vi "MultiChannelfFeedbackCooling (FPGA).vi"() -> ()   [LabVIEW 2016]
doc: "This VI will read single point values from 4 channels of a R Series board at a specified rate."
uses:
  <vilib>/rvi/Emulation/niFpgaGetClockAttributes.vi
  <vilib>/rvi/Emulation/niFpgaSctlEmulationGetInTimedLoop.vi
  <vilib>/rvi/Emulation/niFpgaEmulationReportErrorSimple.vi
  <vilib>/rvi/eio/common/nirviEmuTemplateMethod_errors.vi
  <vilib>/rvi/Memory/Memory_Emulation/nirvimemoryFastEmulation.vi
  <vilib>/rvi/Memory/Memory_Emulation/nirvimemoryEmulation.vi
  <vilib>/rvi/Emulation/niFpgaEmulationIsFPGAContextNoSignature.vi
  <vilib>/rvi/DataTransferAndStorage/Container/Common/niFpgaContainerGetUniqueNameForEmu.vi
  <vilib>/rvi/Emulation/niFpgaProcessEmulError.vi
  <vilib>/rvi/errors/nirviReportUnexpectedCaseInternalError (U32).vi
  <vilib>/rvi/Memory/Memory_Emulation/niFpgaMemoryEmulationCacheClearOnFirstRun.vi
  <vilib>/rvi/Memory/Memory_Emulation/nirvimemoryEmulationManagerCache_MakeExclusive.vi
  <vilib>/rvi/Memory/Memory_Emulation/niFpgaMemoryEmulationValidateCache.vi
  <vilib>/rvi/Memory/Memory_Emulation/nirvimemoryEmulationManagerCache_InsertValue.vi
  <vilib>/Utility/error.llb/Clear Errors.vi
  <vilib>/rvi/Memory/Memory_Emulation/nirvimemoryEmulationManagerCache_ReleaseExclusive.vi
  <vilib>/rvi/Memory/Memory_Emulation/nirvimemoryEmulationManagerCache_GetValue.vi
  <vilib>/rvi/Memory/Memory_Emulation/nirvimemoryEmulationManagerCache_SetValue.vi
  <vilib>/rvi/Emulation/niFpgaSctlEmulationResourceMgr.vi
  <vilib>/rvi/Emulation/niFpgaCriticalErrorInLSC.vi
  <vilib>/eio/EIONode/EIONode.xnode
  <vilib>/rvi/DataTransferAndStorage/Container/XNode/niFpgaContainer.xnode
  <vilib>/rvi/FXPMathLib/FxpInterpret/XNode/nifxpmath_Interpret.xnode
panel:
  in  "pg_img":fxp<+/-,24,12>
  in  "dg_img":fxp<+/-,24,12>
  in  "ig_img":fxp<+/-,24,6>
  in  "setpt_img":i16
  out "AI_img":i16
  in  "lp coeff_img":i32[](array[numeric])=[1008310688, 32715568]
  in  "Upper lim_img":fxp<+/-,16,16>
  in  "Lower lim_img":fxp<+/-,16,16>
  in  "lp coeff d2":i32[](array[numeric])=[1008310688, 32715568]
  in  "hp coeff_img":i32[](array[numeric])=[946630756, 1010186290]
  out "tot_fb_img":i16
  out "fb_img":i16
  in  "output offset_img":i16
  in  "lp coeff 2":i32[](array[numeric])=[1008310688, 32715568]
  in  "data_buffer3":i16
  in  "Arb gain (ch2)":fxp<+/-,24,12>=0.5 caption="RMS"
  in  "lp coeff 0":i32[](array[numeric])=[1008310688, 32715568]
  in  "lp coeff 1":i32[](array[numeric])=[1008310688, 32715568]
  in  "hp coeff d2":i32[](array[numeric])=[946630756, 1010186290]
  in  "hp coeff 2":i32[](array[numeric])=[946630756, 1010186290]
  in  "hp coeff 1":i32[](array[numeric])=[946630756, 1010186290]
  in  "hp coeff 0":i32[](array[numeric])=[946630756, 1010186290]
  in  "Use_PID2_X 2":bool
  out "AI5":i16
  in  "Dc Pos d2":i16
  out "tot_fb_2":i16
  out "tot_fb_1":i16
  out "tot_fb_0":i16
  out "fb_d2":i16
  in  "output offset 2":i16
  in  "output offset 1":i16
  in  "output offset 0":i16
  in  "Lower lim 4":fxp<+/-,16,16>
  in  "Upper lim d0 3":fxp<+/-,16,16>
  in  "pg d0 3":fxp<+/-,24,12>
  in  "ig d03":fxp<+/-,24,6>
  in  "dg d0 3":fxp<+/-,24,12>
  out "fb_2":i16
  in  "ig 3":fxp<+/-,24,6>
  out "written_address":u32
  in  "ready_to_write":bool
  in  "Arb steps per cycle":u16
  in  "data_buffer2":i16
  in  "data_buffer_1":i16
  in  "write_address":u16
  in  "Arb gain (ch1)":fxp<+/-,24,12>=0.5 caption="RMS"
  in  "Arb gain (ch0)":fxp<+/-,24,12>=0.5 caption="RMS"
  out "fb_1":i16
  out "fb_0":i16
  in  "Dc Pos 1":i16
  in  "Dc Pos 0":i16
  in  "Lower lim 2":fxp<+/-,16,16>
  in  "Upper lim 2":fxp<+/-,16,16>
  in  "dg 2":fxp<+/-,24,12>
  in  "pg 2":fxp<+/-,24,12>
  out "AI2":i16
  in  "Dc Pos 2":i16
  out "AI1":i16
  in  "dg 1":fxp<+/-,24,12>
  in  "Upper lim 1":fxp<+/-,16,16>
  in  "Lower lim 1":fxp<+/-,16,16>
  out "AI0":i16
  in  "dg 0":fxp<+/-,24,12>
  in  "Upper lim 0":fxp<+/-,16,16>
  in  "Lower lim 0":fxp<+/-,16,16>
  in  "Count(uSec)":u32
  out "FPGA Error Out":errorcluster
  in  "Stop":bool
  # "test"
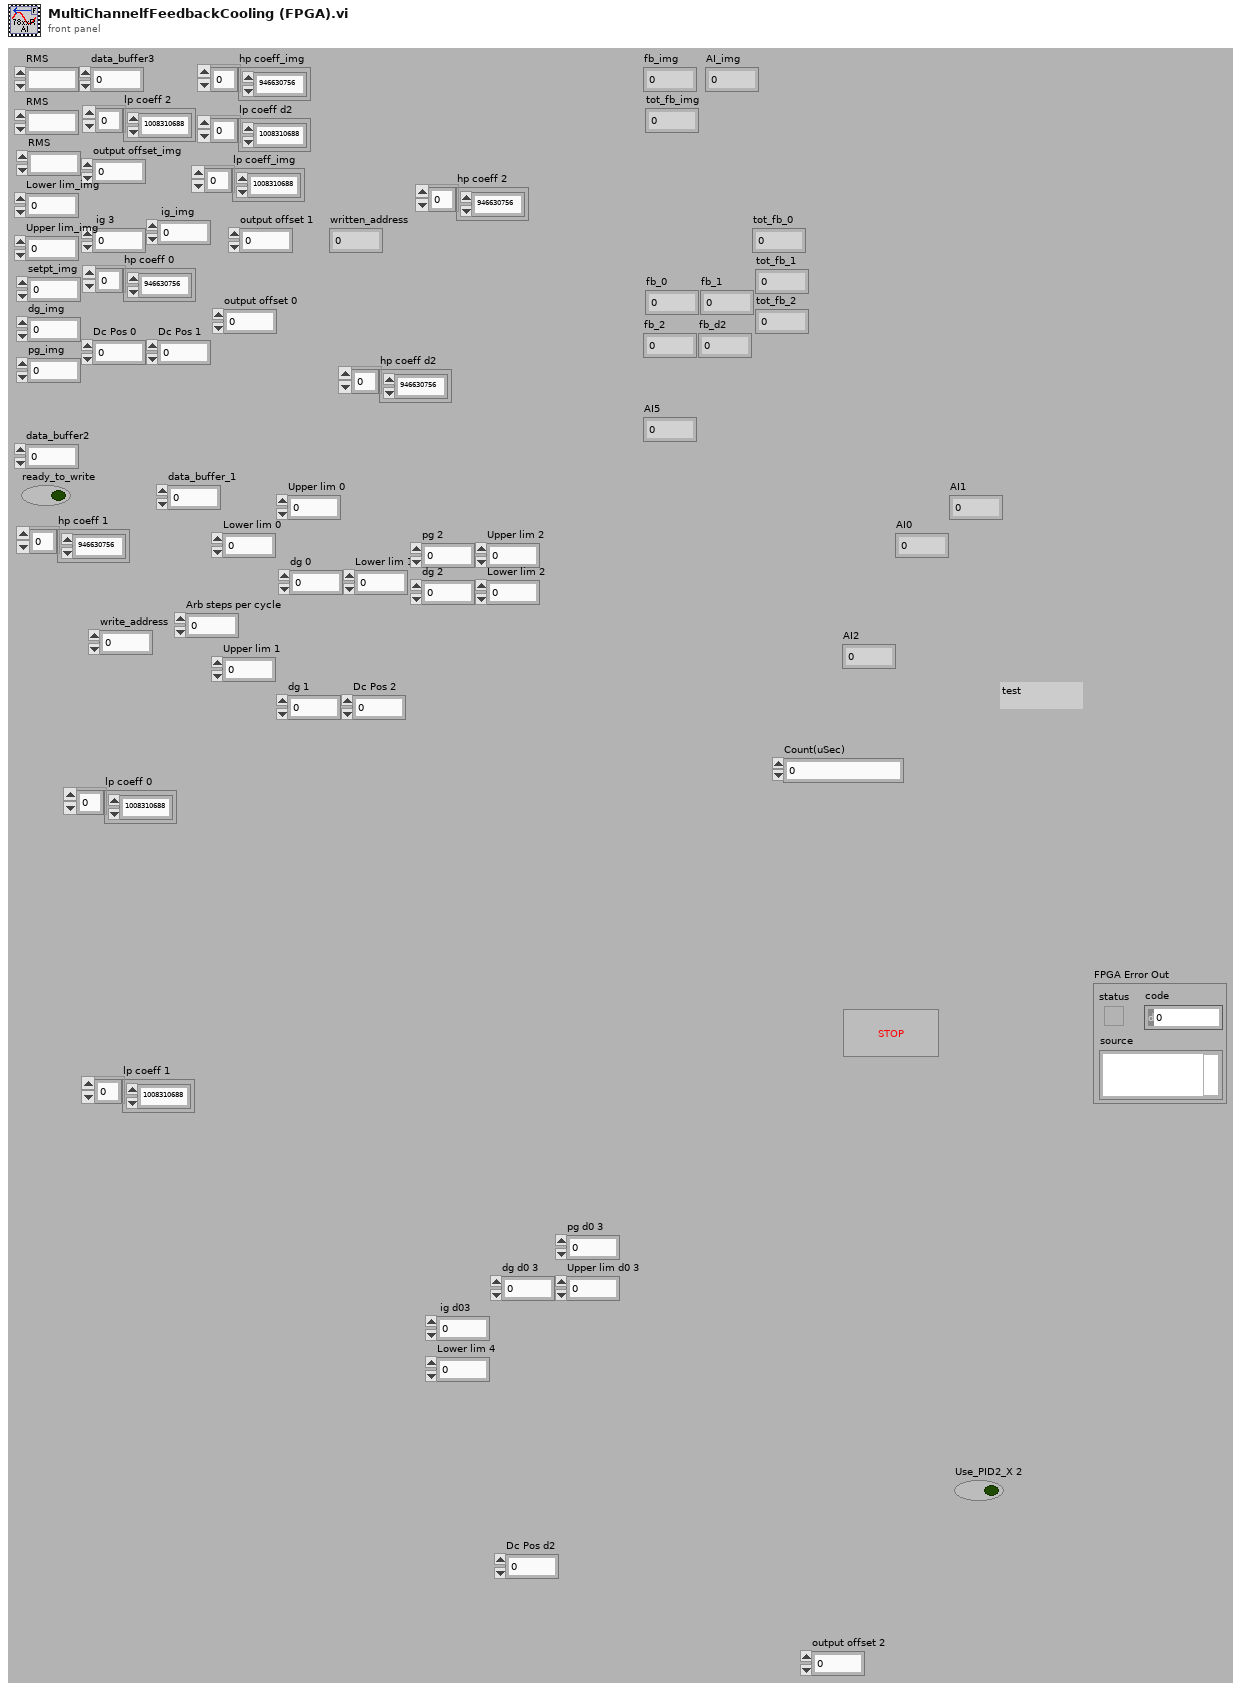
[diagram p1: front panel]
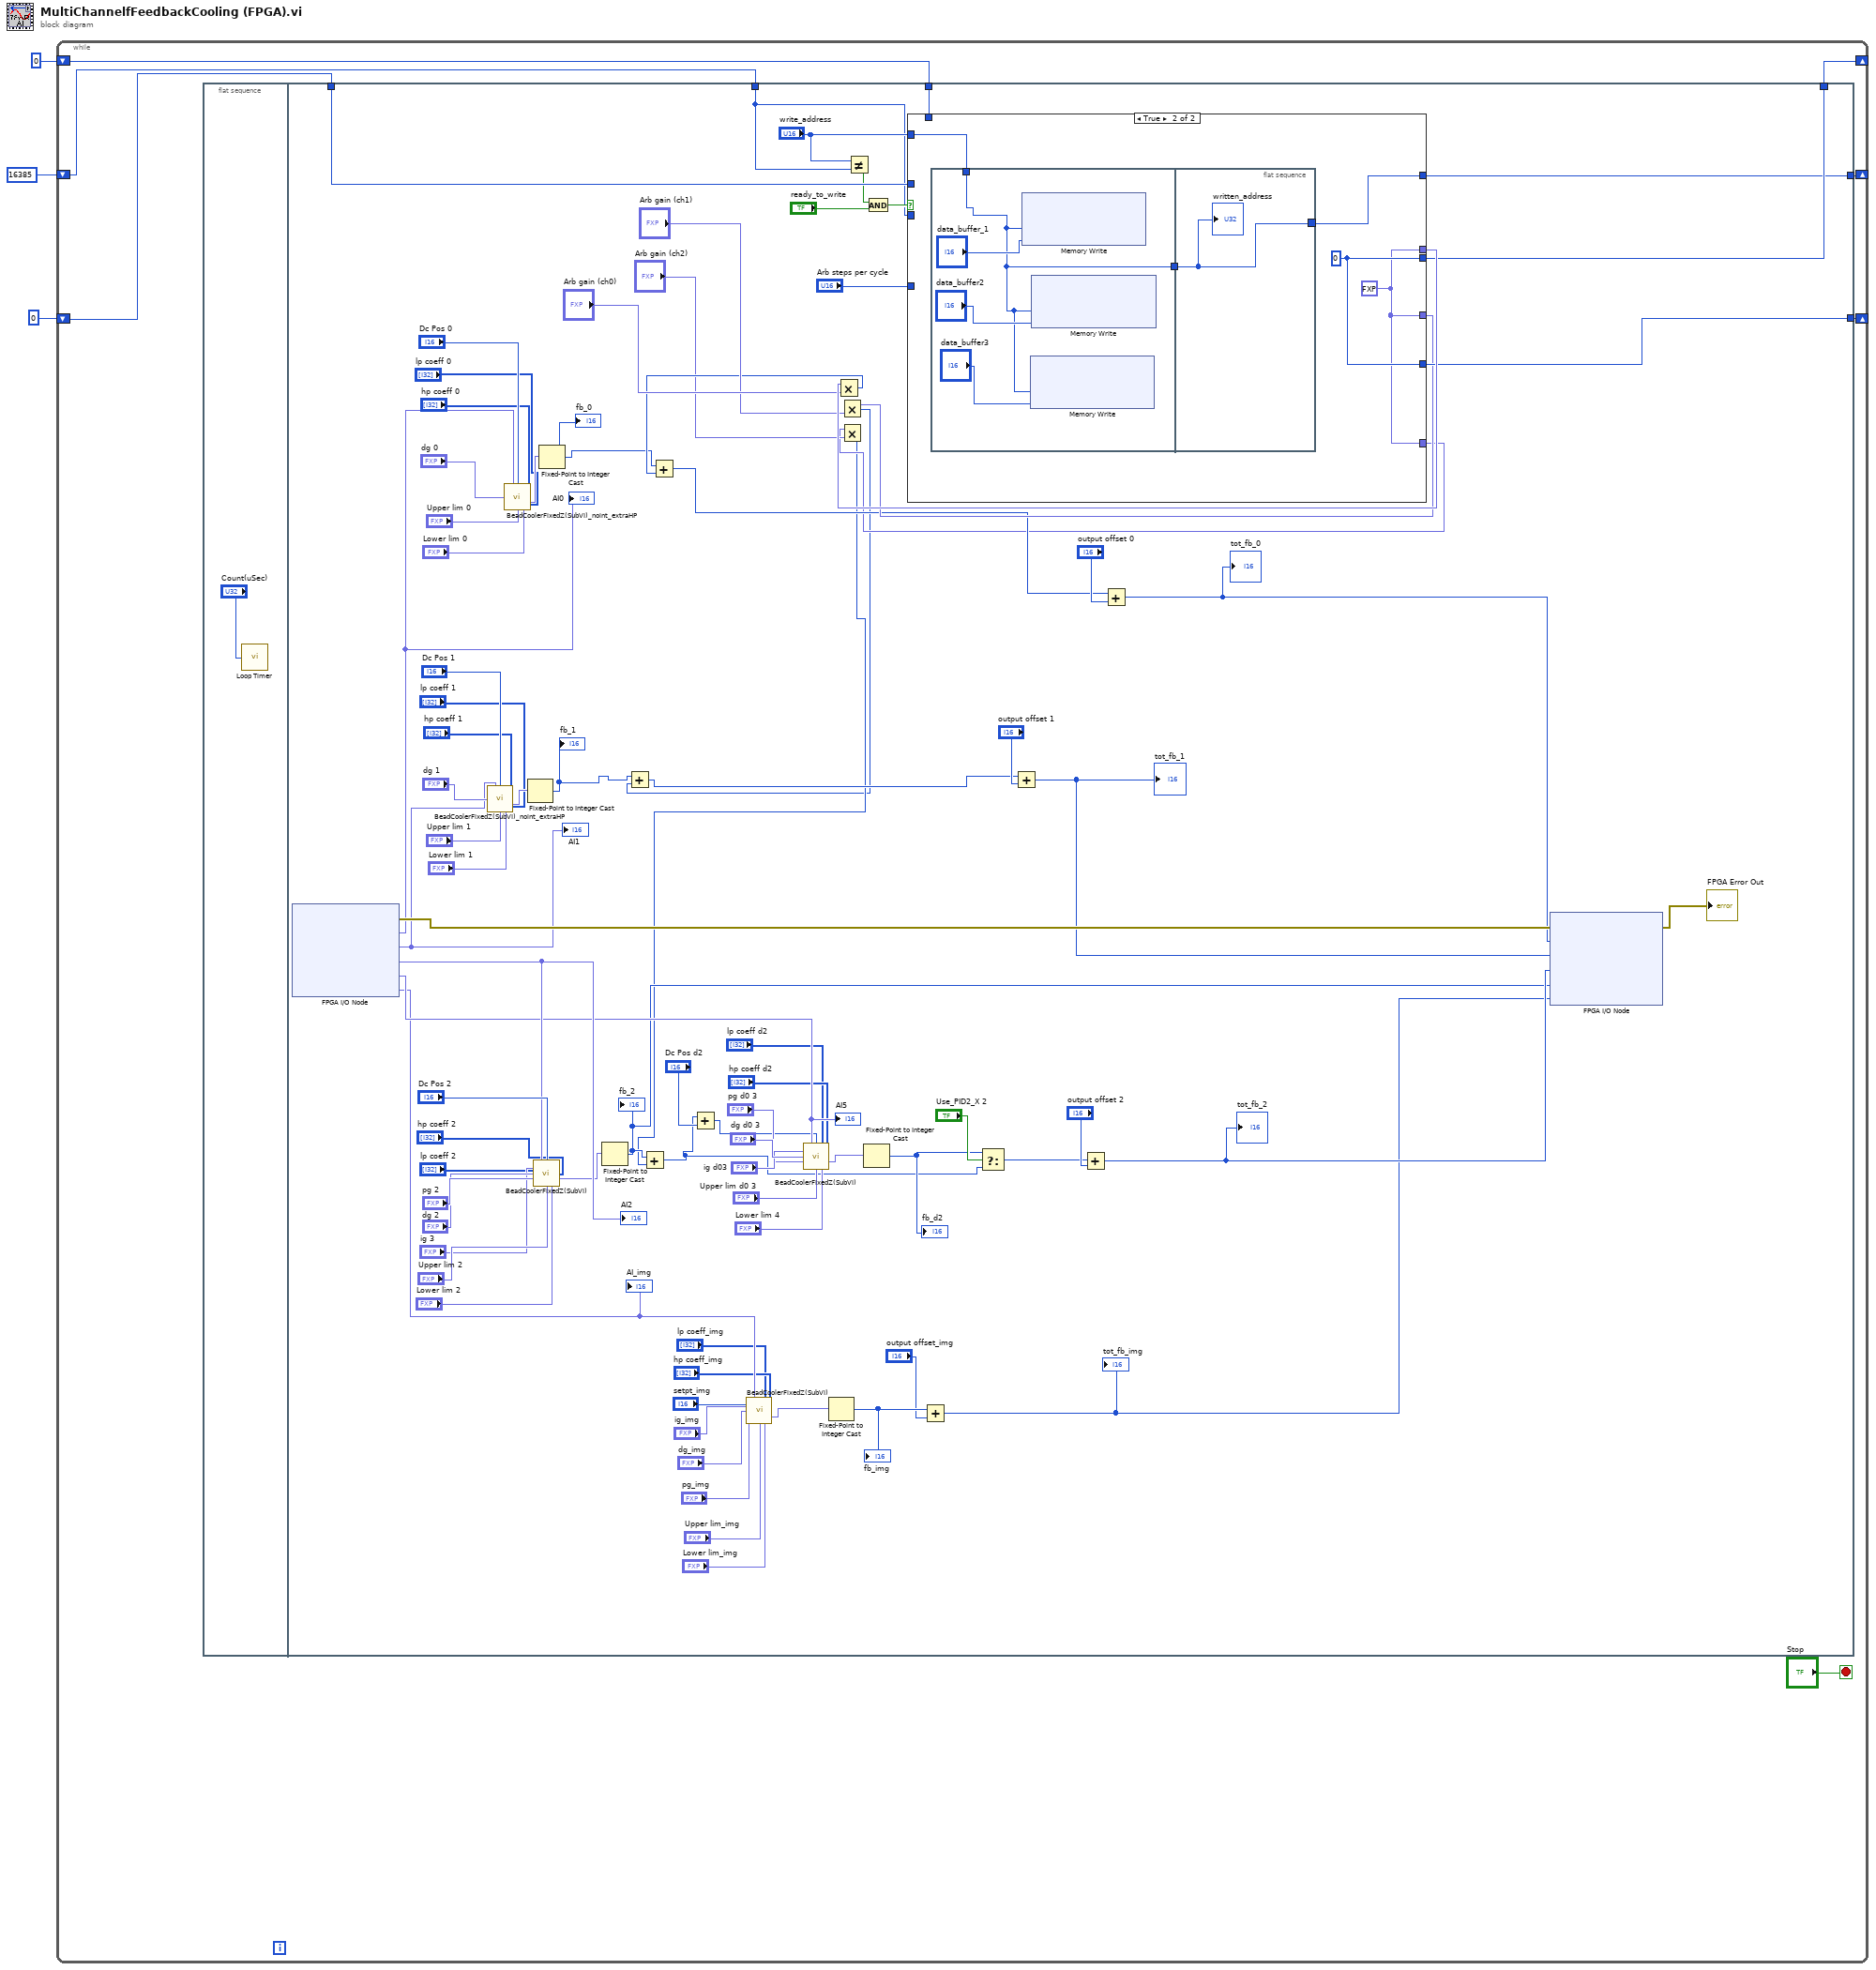
[diagram p0: block diagram]
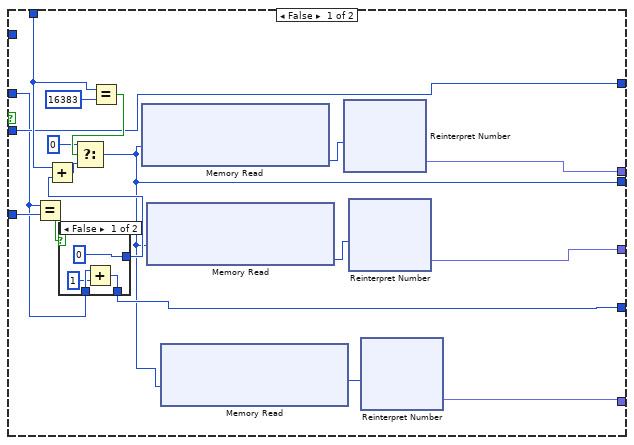
[diagram p2: hidden frame]
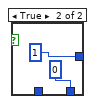
[diagram p3: hidden frame]
diagram:
  n1 = while {
    shift-right: [w9] -> _
    shift-left: u16 0 ("t") -> [w8]
    shift-right: [w7] -> _
    shift-left: u16 0 ("t") -> [w4]
    shift-right: [w6] -> _
    shift-left: u32 16385 ("write_address") -> [w5]
    stop <- "Stop" stop-if-true
    n2 = flat-sequence {
      tunnel: [w81] -> w9
      tunnel: w8 -> [w80]
      tunnel: [w78] -> w7
      tunnel: w4 -> [w77]
      tunnel: [w76] -> w6
      tunnel: w5 -> [w68]
      frame #0 {
        n3 = call "Loop Timer"("Count(uSec)"="Count(uSec)") -> ()  [unwired: 1 out]
      }
      frame #1 {
        n4 = xnode "FPGA I/O Node"() -> ("error out"=w98:errorcluster, "Connector0/AI0"=w67:fxp<+/-,27,5>, "Connector0/AI1"=w66:fxp<+/-,27,5>, "Connector0/AI2"=w63:fxp<+/-,27,5>, "Connector0/AI5"=w51:fxp<+/-,27,5>, "Connector0/AI4"=w25:fxp<+/-,27,5>)  [unwired: 6 in, 5 out]
        "AI0" <- w67
        "AI1" <- w66
        "AI2" <- w63
        "AI5" <- w51
        "AI_img" <- w25
        n5 = call "BeadCoolerFixedZ(SubVI)_noint_extraHP.vi"("AI0"=w66, "Dc Pos"="Dc Pos 1", "dg"="dg 1", "hp coeff"="hp coeff 1", "lp coeff"="lp coeff 1", "Upper lim"="Upper lim 1", "Lower lim"="Lower lim 1") -> ("Output"=w65:fxp<+/-,16,16>)  [unwired: 8 in]
        n6 = call "BeadCoolerFixedZ(SubVI)_noint_extraHP.vi"("AI0"=w67, "Dc Pos"="Dc Pos 0", "dg"="dg 0", "hp coeff"="hp coeff 0", "lp coeff"="lp coeff 0", "Upper lim"="Upper lim 0", "Lower lim"="Lower lim 0") -> ("Output"=w69:fxp<+/-,16,16>)  [unwired: 8 in]
        n7 = Fixed-Point to Integer Cast(1:w65) -> (0:w30:i16)
        "fb_1" <- w30
        n8 = call "BeadCoolerFixedZ(SubVI).vi"("AI0"=w63, "Dc Pos"="Dc Pos 2", "lp coeff"="lp coeff 2", "ig"="ig 3", "dg"="dg 2", "hp coeff"="hp coeff 2", "pg"="pg 2", "Upper lim"="Upper lim 2", "Lower lim"="Lower lim 2") -> ("Output"=w39:fxp<+/-,16,16>)  [unwired: 6 in]
        n9 = Fixed-Point to Integer Cast(1:w69) -> (0:w33:i16)
        "fb_0" <- w33
        n10 = Fixed-Point to Integer Cast(1:w39) -> (0:w34:i16)
        "fb_2" <- w34
        n11 = call "BeadCoolerFixedZ(SubVI).vi"("AI0"=w25, "Dc Pos"="setpt_img", "lp coeff"="lp coeff_img", "ig"="ig_img", "dg"="dg_img", "hp coeff"="hp coeff_img", "pg"="pg_img", "Upper lim"="Upper lim_img", "Lower lim"="Lower lim_img") -> ("Output"=w24:fxp<+/-,16,16>)  [unwired: 6 in]
        n12 = Fixed-Point to Integer Cast(1:w24) -> (0:w23:i16)
        "fb_img" <- w23
        n13 = Not Equal?(x="write_address", y=w68) -> (x != y?=w73:bool)
        n14 = And(x=w73, y="ready_to_write") -> (x .and. y?=w74:bool)
        n15 = case shown="True" w74 {
          tunnel: [w115 w123] -> w83
          tunnel: [w100 w127] -> w81
          tunnel: w80 -> [w108 _]
          tunnel: [w109 w123] -> w71
          tunnel: "Arb steps per cycle" -> [w107 _]
          tunnel: [w102 w127] -> w78
          tunnel: w77 -> [w103 _]
          tunnel: [w106 w125] -> w76
          tunnel: w68 -> [w106 _]
          tunnel: "write_address" -> [_ w124]
          tunnel: [w99 w123] -> w31
          frame False {
            n16 = Equal?(x=w103, y=w107) -> (x = y?=w105:bool)
            n17 = case shown="False" w105 {
              tunnel: [u16 0 ("y") u16 1 ("y")] -> w104
              tunnel: w103 -> [w119 _]
              tunnel: [w117 u16 0] -> w102
              frame False {
                n18 = Add(x=w119, y=u16 1) -> (x+y=w117:u16)
              }
              frame True {
              }
            }
            n19 = Add(x=w108, y=w104) -> (x+y=w111:u16)
            n20 = Equal?(x=w108, y=u16 16383) -> (x = y?=w113:bool)
            n21 = Select(t=u16 0, s=w113, f=w111) -> (s? t:f=w100:u16)
            n22 = xnode ("Memory Read")("Address"=w100) -> ("Data"=w116:i16)  [unwired: 1 in, 1 out]
            n23 = xnode ("Memory Read")("Address"=w100) -> ("Data"=w110:i16)  [unwired: 1 in, 1 out]
            n24 = xnode ("Memory Read")("Address"=w100) -> ("Data"=w101:i16)  [unwired: 1 in, 1 out]
            n25 = xnode "Reinterpret Number"("x"=w116) -> ("y"=w115:fxp<+/-,16,16>)
            n26 = xnode "Reinterpret Number"("x"=w110) -> ("y"=w109:fxp<+/-,16,16>)
            n27 = xnode "Reinterpret Number"("x"=w101) -> ("y"=w99:fxp<+/-,16,16>)
          }
          frame True {
            w127 = u16 0
            w123 = fxp<+/-,16,16> 0.0 ("y")
            n28 = flat-sequence {
              tunnel: [w129] -> w126
              tunnel: w124 -> [w129]
              tunnel: w126 -> [w132]
              tunnel: [w132] -> w125
              frame #0 {
                n29 = xnode ("Memory Write")("Address"=w129, "Data"="data_buffer_1") -> ()  [unwired: 1 in, 1 out]
                n30 = xnode ("Memory Write")("Address"=w129, "Data"="data_buffer3") -> ()  [unwired: 1 in, 1 out]
                n31 = xnode ("Memory Write")("Address"=w129, "Data"="data_buffer2") -> ()  [unwired: 1 in, 1 out]
              }
              frame #1 {
                "written_address" <- w132
              }
            }
          }
        }
        n32 = Multiply(x=w83, y="Arb gain (ch0)") -> (x*y=w55:i16)
        n33 = Add(x=w33, y=w55) -> (x+y=w44:i16)
        n34 = Multiply(x=w71, y="Arb gain (ch1)") -> (x*y=w27:i16)
        n35 = Add(x=w30, y=w27) -> (x+y=w29:i16)
        n36 = Multiply(x=w31, y="Arb gain (ch2)") -> (x*y=w28:i16)
        n37 = Add(x=w34, y=w28) -> (x+y=w38:i16)
        n38 = Add(x=w38, y="Dc Pos d2") -> (x+y=w35:i16)
        n39 = call "BeadCoolerFixedZ(SubVI).vi"("AI0"=w51, "Dc Pos"=w35, "lp coeff"="lp coeff d2", "ig"="ig d03", "dg"="dg d0 3", "hp coeff"="hp coeff d2", "pg"="pg d0 3", "Upper lim"="Upper lim d0 3", "Lower lim"="Lower lim 4") -> ("Output"=w57:fxp<+/-,16,16>)  [unwired: 6 in]
        n40 = Fixed-Point to Integer Cast(1:w57) -> (0:w47:i16)
        "fb_d2" <- w47
        n41 = Add(x=w23, y="output offset_img") -> (x+y=w22:i16)
        "tot_fb_img" <- w22
        n42 = Select(t=w47, s="Use_PID2_X 2", f=w38) -> (s? t:f=w46:i16)
        n43 = Add(x=w29, y="output offset 1") -> (x+y=w48:i16)
        "tot_fb_1" <- w48
        n44 = Add(x=w46, y="output offset 2") -> (x+y=w45:i16)
        "tot_fb_2" <- w45
        n45 = Add(x=w44, y="output offset 0") -> (x+y=w49:i16)
        "tot_fb_0" <- w49
        n46 = xnode "FPGA I/O Node"("error in"=w98, "Connector0/AO0"=w49, "Connector0/AO1"=w48, "Connector0/AO2"=w45, "Connector0/AO3"=w34, "Connector0/AO4"=w22) -> ("error out"=→"FPGA Error Out":errorcluster)  [unwired: 5 in, 5 out]
      }
    }
  }
